vi "GitCheckoutByHash.vi"(8 "error in (no error)":errorcluster, 9 "File":path=path "", 10 "Hash":string, 11 "Git exec":string="git") -> (0 "error out":errorcluster, 1 "File out":path, 2 "Response":string, 3 "Git exec out":string="git")   [LabVIEW 2013]
uses:
  GitCmd.vi
  <vilib>/dlg_ctls.llb/Space Constant.vi
  <vilib>/Platform/system.llb/System Exec.vi
  <vilib>/Utility/error.llb/Error Cluster From Error Code.vi
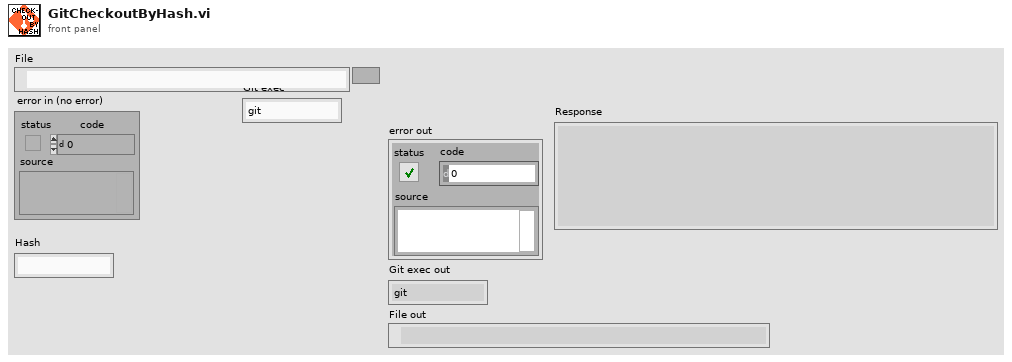
[diagram p1: front panel]
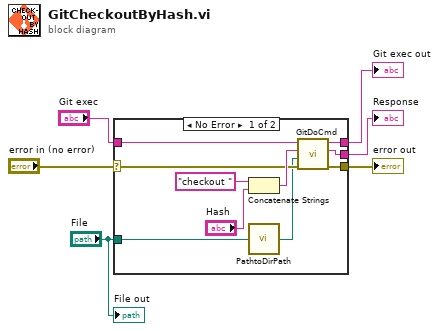
[diagram p0: block diagram]
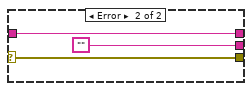
[diagram p2: hidden frame]
diagram:
  n1 = case shown="No Error" "error in (no error)" {
    selector: "error in (no error)" -> [w11 w18]
    tunnel: "Git exec" -> [w15 w17]
    tunnel: "File" -> [w8 _]
    tunnel: [w12 ""] -> w4
    tunnel: [w10 w18] -> w3
    tunnel: [w13 w17] -> w1
    frame No Error {
      n2 = Concatenate Strings("checkout " ("string"), "Hash") -> (w14:string)
      n3 = call "PathtoDirPath.vi"("Path"=w8) -> ("Path out"=w7:path)
      n4 = call "GitDoCmd.vi"("error in (no error)"=w11, "Working Path"=w7, "Git command"=w14, "Git exec"=w15) -> ("error out"=w10:errorcluster, "Returned stdout"=w12:string, "Git exec out"=w13:string)  [unwired: 3 in, 1 out]
    }
    frame Error {
    }
  }
  "Response" <- w4
  "error out" <- w3
  "Git exec out" <- w1
  "File out" <- "File"
